vi "Generate Data.vi"(8 "Error In":errorcluster, 11 "String in":refnum<class "String.lvclass">) -> (0 "Error Out":errorcluster, 3 "String out":refnum<class "String.lvclass">)   [LabVIEW 2023, in "String.lvclass"]
doc: "The method generates random string data to be transmitted."
uses:
  String.lvclass
  C:/Users/Ancy.Augustin/Downloads/Messenger/Messenger/Classes/Data/Data.lvclass
  String.lvclass/String.ctl
  Display Data.vi
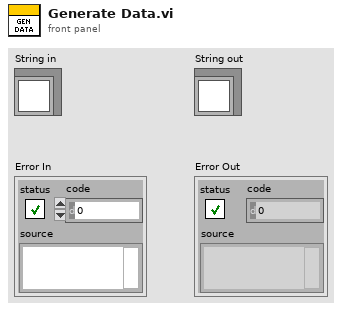
[diagram p1: front panel]
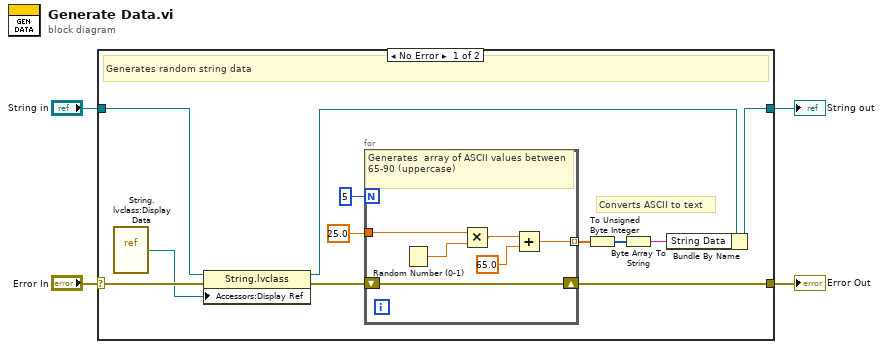
[diagram p0: block diagram]
diagram:
  n1 = case shown="No Error" "Error In" {
    selector: "Error In" -> [w16 w24]
    tunnel: [w15 w24] -> w3
    tunnel: [w10 w23] -> w1
    tunnel: "String in" -> [w7 w23]
    frame No Error {
      # "Converts ASCII to text"
      # "Generates random string data"
      n2 = vi-ref "String.lvclass:Display Data.vi"() -> (w5:refnum<vi>)
      n3 = property class="String.lvclass"(reference=w7, error in=w16, "Accessors:Display Ref"=w5) -> (reference out=w6:refnum<class "String.lvclass">, error out=w8:errorcluster)
      n4 = for {
        N: 5 -> [_]
        shift-right: [w22] -> w15
        shift-left: w8 -> [w22]
        tunnel: 25.0 -> [w20]
        tunnel: [w17] -> w12 mode=indexing
        # "Generates  array of ASCII values between 65-90 (uppercase)"
        n5 = Random Number (0-1)() -> (number: 0 to 1=w21:dbl)
        n6 = Multiply(x=w20, y=w21) -> (x*y=w19:dbl)
        n7 = Add(x=w19, y=65.0) -> (x+y=w17:dbl)
      }
      n8 = To Unsigned Byte Integer(number=w12) -> (unsigned 8bit integer=w11:u8[])
      n9 = Byte Array To String(unsigned byte array=w11) -> (string=w9:string)
      n10 = Bundle By Name(cluster=w6, "String Data"=w9) -> (w10:refnum<class "String.lvclass">)
    }
    frame Error {
    }
  }
  "Error Out" <- w3
  "String out" <- w1
